vi "Scale.vi"(8 "error in (no error)":errorcluster, 10 "Waveform in":waveform(dbl)[](array[waveform]), 11 "NI_DAQmx(AI) in":refnum<class "NI_DAQmx(AI).lvclass">) -> (0 "error out":errorcluster, 2 "Waveform out":waveform(dbl)[](array[waveform]), 3 "NI_DAQmx(AI) out":refnum<class "NI_DAQmx(AI).lvclass">)   [LabVIEW 2025, in "NI_DAQmx(AI).lvclass"]
uses:
  NI_DAQmx(AI).lvclass
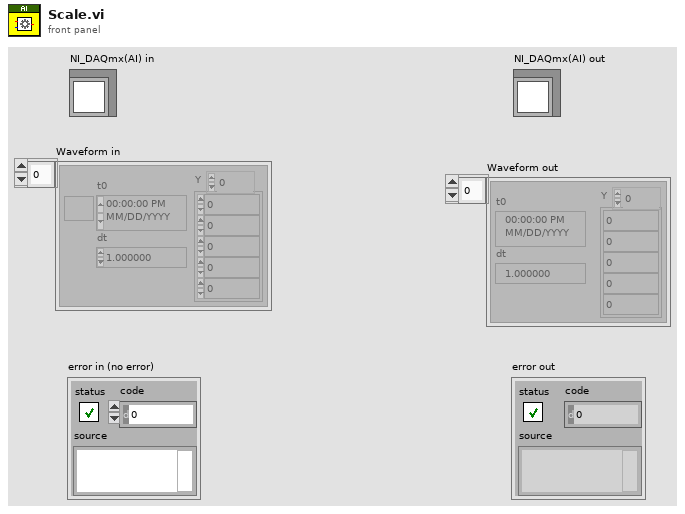
[diagram p1: front panel]
types:
  T1 = typedef "DAQ_Module.lvlib/DAQ_Module.lvclass/DAQ_AI_Task_Config.ctl" = cluster{"AI":cluster{"MaxValue":dbl, "MinValue":dbl, "InputTerminalConfiguration":i32}, "Scale":cluster{"Offset":dbl, "Gain":dbl, "Unit":string}, "Calibrate":cluster{"K":dbl, "B":dbl}}
  T2 = map{string, cluster{"Name":string, "Data out":T1}}
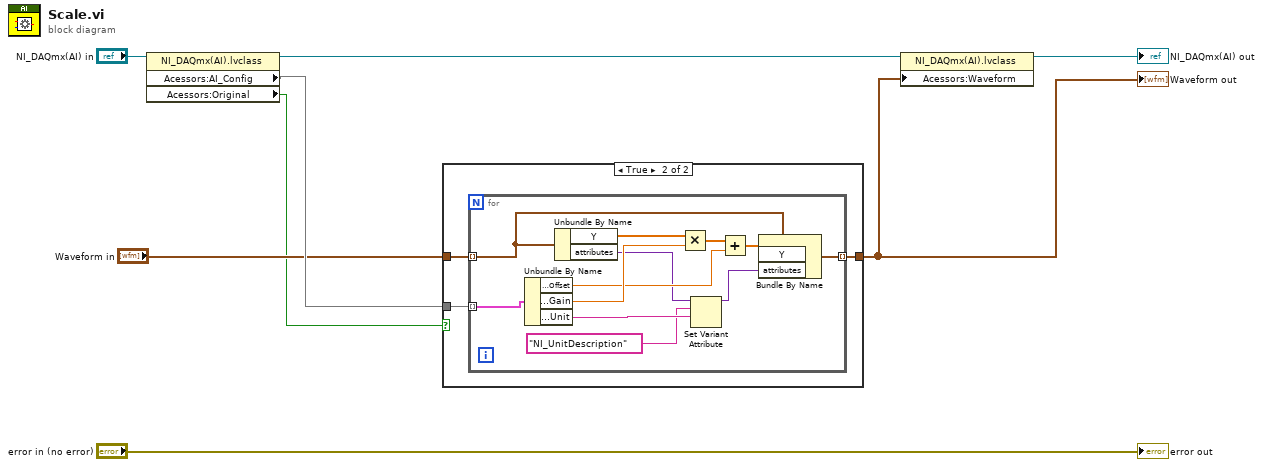
[diagram p0: block diagram]
diagram:
  n1 = property class="NI_DAQmx(AI).lvclass"(reference="NI_DAQmx(AI) in") -> (reference out=w6:refnum<class "NI_DAQmx(AI).lvclass">, "Acessors:AI_Config"=w5:T2, "Acessors:Original"=w1:bool)  [unwired: 1 in, 1 out]
  n2 = case shown="True" w1 {
    tunnel: "Waveform in" -> [w9 w12]
    tunnel: w5 -> [_ w11]
    tunnel: [w9 w10] -> w2
    frame False {
    }
    frame True {
      n3 = for {
        tunnel: w12 -> [w19] mode=indexing
        tunnel: w11 -> [w23] mode=indexing
        tunnel: [w13] -> w10 mode=indexing
        n4 = Unbundle By Name(w23) -> ("Config.Data out.Scale.Offset"=w20:dbl, "Config.Data out.Scale.Gain"=w22:dbl, "Config.Data out.Scale.Unit"=w15:string)
        n5 = Unbundle By Name(w19) -> ("Y"=w24:dbl[], "attributes"=w17:variant)
        n6 = Multiply(x=w24, y=w22) -> (x*y=w21:dbl[])
        n7 = Set Variant Attribute(Variant=w17, name="NI_UnitDescription", value=w15) -> (Variant out=w16:variant)  [unwired: 1 in, 2 out]
        n8 = Add(x=w21, y=w20) -> (x+y=w18:dbl[])
        n9 = Bundle By Name(cluster=w19, "Y"=w18, "attributes"=w16) -> (w13:waveform(dbl))
      }
    }
  }
  "Waveform out" <- w2
  n10 = property class="NI_DAQmx(AI).lvclass"(reference=w6, "Acessors:Waveform"=w2) -> (reference out=→"NI_DAQmx(AI) out":refnum<class "NI_DAQmx(AI).lvclass">)  [unwired: 1 in, 1 out]
  "error out" <- "error in (no error)"
